vi "Main.vi"() -> ()   [LabVIEW 2015]
doc: "本模板用于队列消息处理器设计模式。\n\n事件处理循环负责按用户界面操作生成对应的消息。\n\n消息处理循环负责对事件处理循环或其他消息生成的消息进行处理。消息内容为字符串值，因此很容易将新消息添加至“消息处理”循环的“消息分支”条件结构。每个消息簇还可选择性地为消息数据提供一个变体，变体数据可以转换为消息数据所需要的任意类型。"
uses:
  State.ctl
  Browse/Browse.lvlib
  Sample/Sample.lvlib
  Debug/Debug.lvlib
panel:
  in  "停止按钮":bool
  in  "Engineering":bool
  in  "Sample":bool
  in  "Browse":bool
  # "WJ90000测量系统"
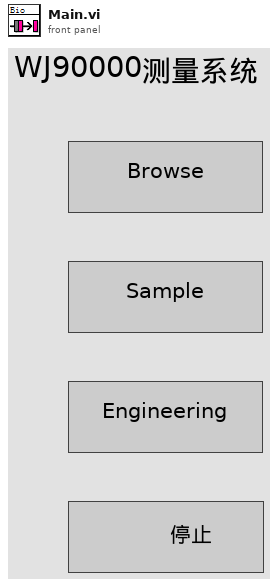
[diagram p1: front panel]
types:
  T1 = typedef "State.ctl" = enum16{"Initialize", "Browse", "Sample", "Engineering", "Wait For Event", "Exit"}
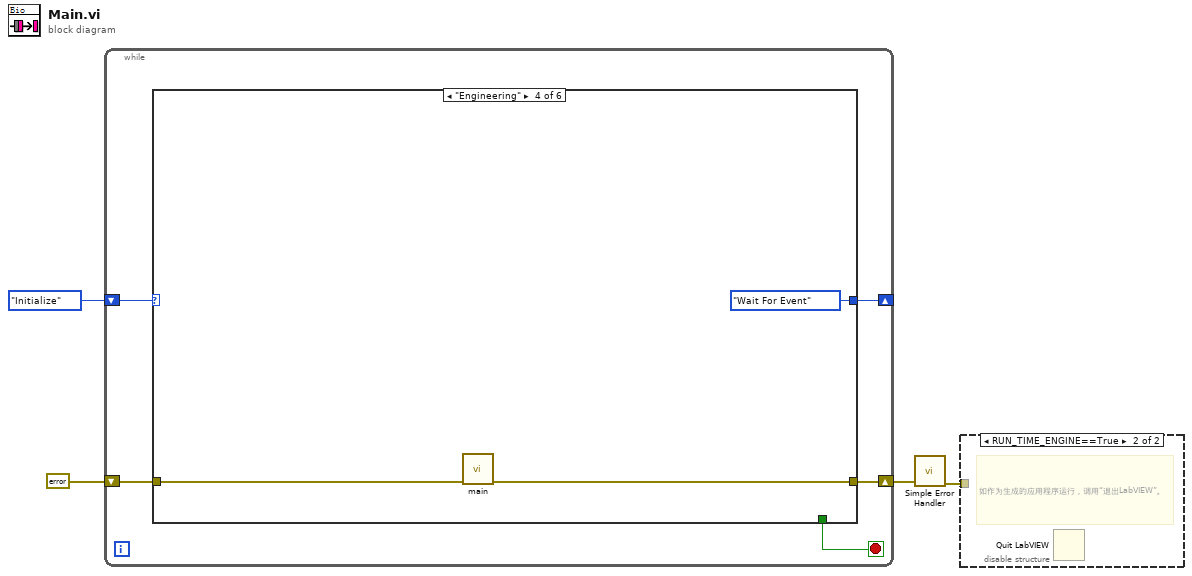
[diagram p0: block diagram]
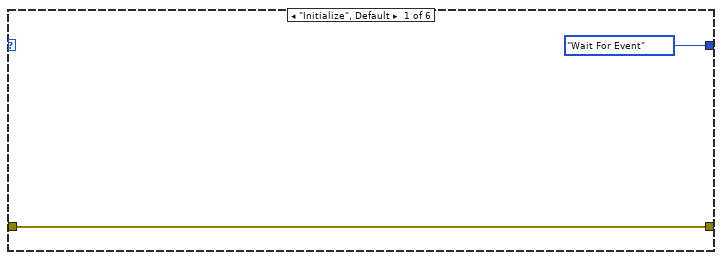
[diagram p2: hidden frame]
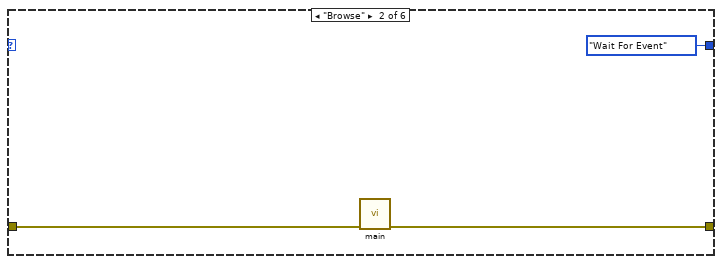
[diagram p3: hidden frame]
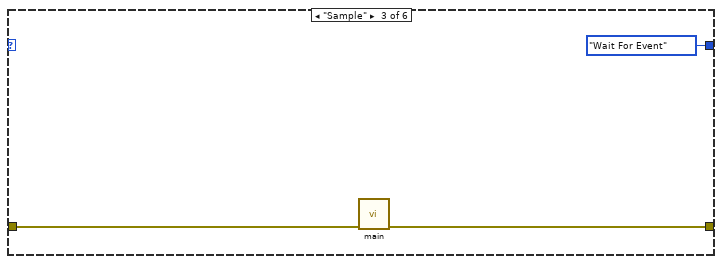
[diagram p4: hidden frame]
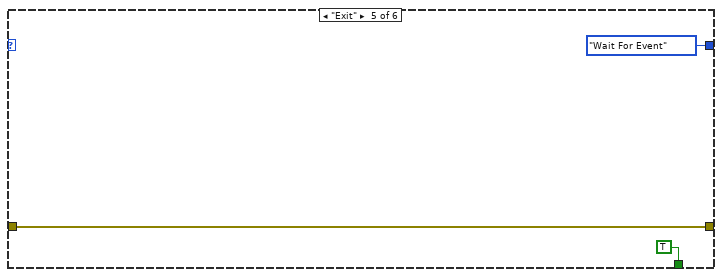
[diagram p5: hidden frame]
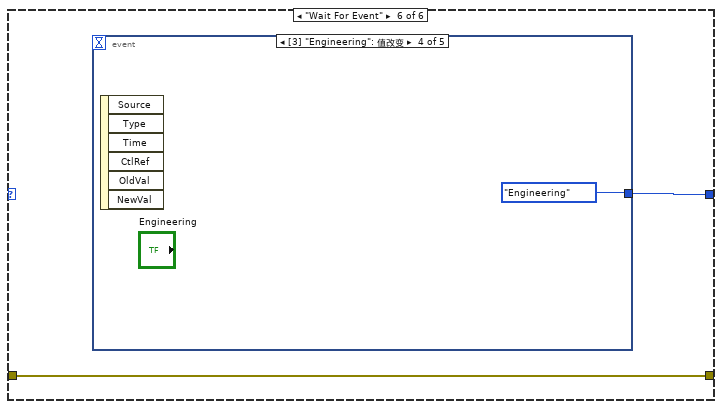
[diagram p6: hidden frame]
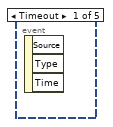
[diagram p7: hidden frame]
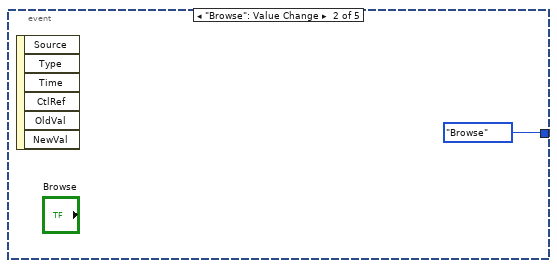
[diagram p8: hidden frame]
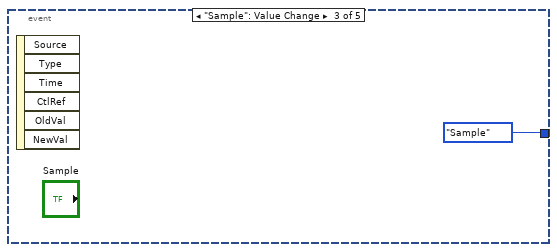
[diagram p9: hidden frame]
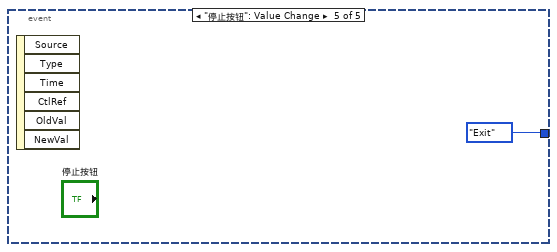
[diagram p10: hidden frame]
diagram:
  n1 = while {
    shift-right: [w8] -> _
    shift-left: State."Initialize" ("State") -> [w9]
    shift-right: [w6] -> w2
    shift-left: errorcluster {"status"=FALSE, "code"=0, "source"=""} ("error out") -> [w7]
    stop <- w5 stop-if-true
    n2 = case shown="\"Engineering\"" w9 {
      tunnel: [State."Wait For Event" ("State") State."Wait For Event" ("State") State."Wait For Event" ("State") State."Wait For Event" ("State") State."Wait For Event" ("State") w25] -> w8
      tunnel: w7 -> [w10 w13 w16 w19 w22 w24]
      tunnel: [w10 w12 w15 w18 w22 w24] -> w6
      tunnel: [_ _ _ _ TRUE _] -> w5
      frame "Initialize", Default {
      }
      frame "Browse" {
        n3 = call "main.vi"("错误常量"=w13) -> ("error out"=w12:errorcluster)  [unwired: 10 in]
      }
      frame "Sample" {
        n4 = call "main.vi"("error in (no error)"=w16) -> ("error out"=w15:errorcluster)  [unwired: 10 in]
      }
      frame "Engineering" {
        n5 = call "main.vi"("error in"=w19) -> ("error out"=w18:cluster{"状态":bool, "代码":i32, "源":string})  [unwired: 10 in]
      }
      frame "Exit" {
      }
      frame "Wait For Event" {
        n6 = event shown="[3] \"Engineering\": 值改变" {
          selector: _ -> [_ _ _ _ _]
          dyn-events: _ -> [_ _ _ _ _]
          timeout: _ -> [_ _ _ _ _]
          tunnel: [_ State."Browse" ("State") State."Sample" ("State") State."Engineering" ("State") State."Exit" ("State")] -> w25
          event Timeout {
            n7 = event-data() -> ()  [unwired: 1 in, 3 out]
          }
          event "Browse": Value Change {
            n8 = event-data() -> ()  [unwired: 1 in, 6 out]
          }
          event "Sample": Value Change {
            n9 = event-data() -> ()  [unwired: 1 in, 6 out]
          }
          event "Engineering": Value Change {
            n10 = event-data() -> ()  [unwired: 1 in, 6 out]
          }
          event "停止按钮": Value Change {
            n11 = event-data() -> ()  [unwired: 1 in, 6 out]
          }
        }
      }
    }
  }
  n12 = call <vilib>:"Simple Error Handler.vi"("error in (no error)"=w2) -> ("error out"=w1:errorcluster)  [unwired: 4 in, 4 out]
  n13 = disable-structure "Conditional Disable Structure" shown="RUN_TIME_ENGINE==True" {
    disable-tunnel: w1 -> [_ _]
    frame condition #0 (active) {
    }
    frame condition #1 {
      # "如作为生成的应用程序运行，调用“退出LabVIEW”。"
      n14 = Quit LabVIEW() -> ()  [unwired: 1 in]
    }
  }
